vi "EF_GetFeaturesVectorPowerSpectrum.vi"(8 "error in (no error)":errorcluster, 11 "Array Of Waveforms in":waveform(dbl)[](array[waveform])) -> (0 "error out":errorcluster, 3 "Features Array out":dbl[][](array[numeric]))   [LabVIEW 2016, in "Feature Extraction.lvlib"]
uses:
  <vilib>/Analysis/2dsp.llb/Power Spectrum (DBL).vi
  Feature Extraction.lvlib
  <vilib>/Analysis/NI_AALPro.lvlib
panel:
  # "This VI is a part of BCI Design library, http://www.ru-bci.org \nCopyright © 2020, Sotnikov Peter, All rights reserved. License: GNU GPLv3"
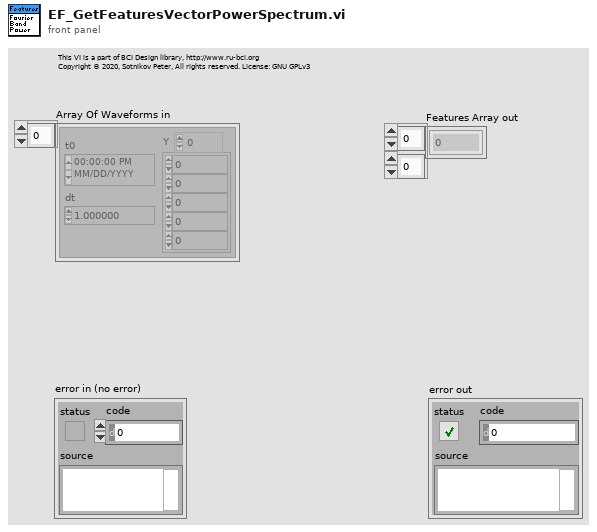
[diagram p1: front panel]
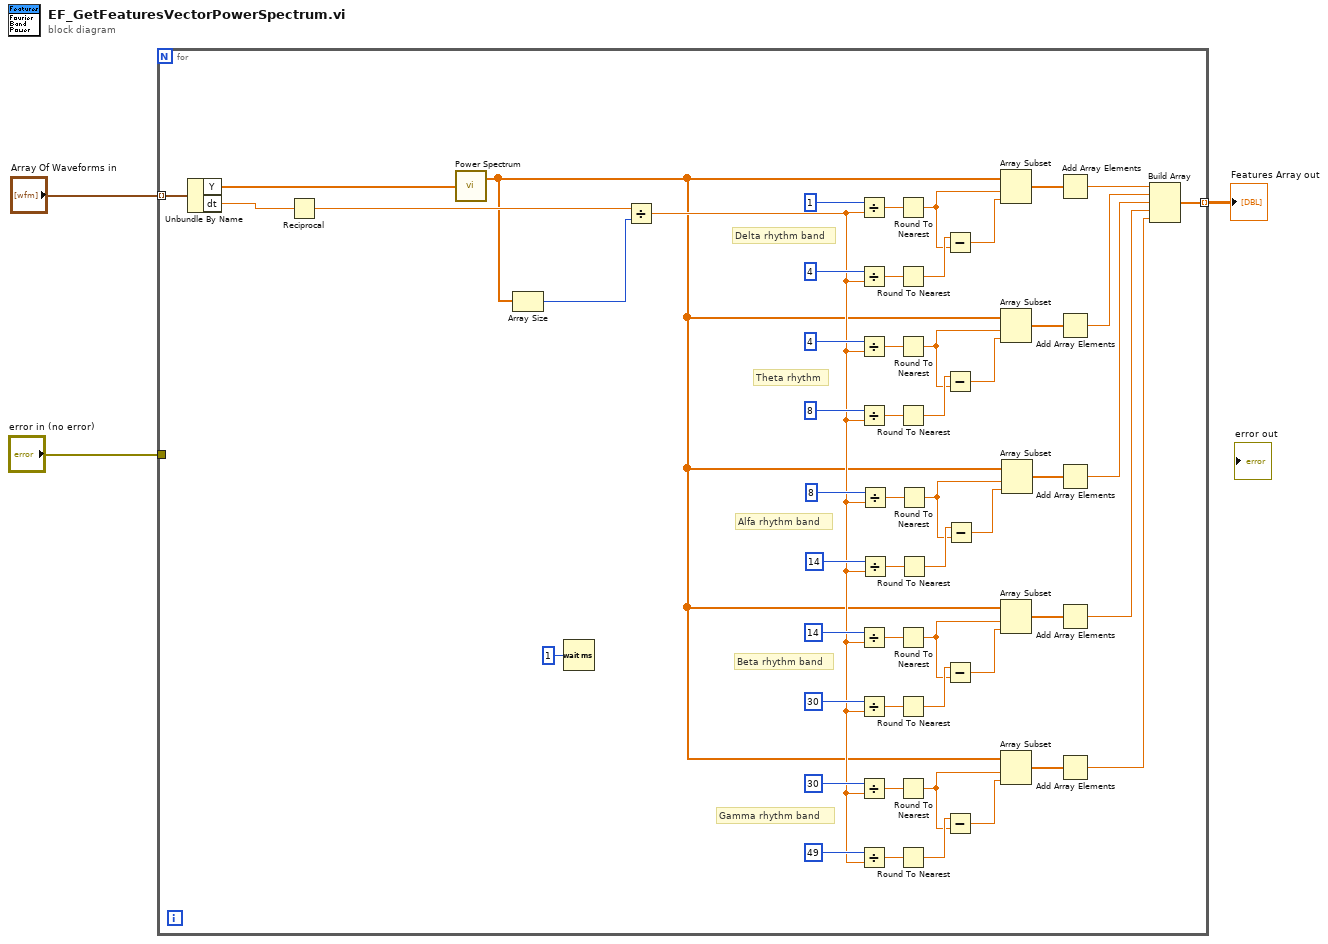
[diagram p0: block diagram]
diagram:
  n1 = for {
    tunnel: "Array Of Waveforms in" -> [w32] mode=indexing
    tunnel: "error in (no error)" -> [_]
    tunnel: [w5] -> w1 mode=indexing
    # "Gamma rhythm band"
    # "Beta rhythm band"
    # "Theta rhythm"
    # "Delta rhythm band"
    # "Alfa rhythm band"
    n2 = Unbundle By Name(w32) -> ("Y"=w4:dbl[], "dt"=w16:dbl)
    n3 = Reciprocal(x=w16) -> (1/x=w7:dbl)
    n4 = call-poly <vilib>:"Power Spectrum.vi"("X"=w4) -> ("Power Spectrum"=w6:dbl[])  [unwired: 1 out]
    n5 = Array Size(array=w6) -> (size(s)=w13:i32)
    n6 = Wait (ms)(milliseconds to wait=u32 1) -> ()  [unwired: 1 out]
    n7 = Divide(x=w7, y=w13) -> (x/y=w15:dbl)
    n8 = Divide(x=1, y=w15) -> (x/y=w57:dbl)
    n9 = Divide(x=4, y=w15) -> (x/y=w55:dbl)
    n10 = Divide(x=4, y=w15) -> (x/y=w52:dbl)
    n11 = Divide(x=8, y=w15) -> (x/y=w50:dbl)
    n12 = Divide(x=14, y=w15) -> (x/y=w42:dbl)
    n13 = Divide(x=30, y=w15) -> (x/y=w40:dbl)
    n14 = Divide(x=30, y=w15) -> (x/y=w37:dbl)
    n15 = Divide(x=49, y=w15) -> (x/y=w35:dbl)
    n16 = Divide(x=8, y=w15) -> (x/y=w47:dbl)
    n17 = Divide(x=14, y=w15) -> (x/y=w45:dbl)
    n18 = Round To Nearest(number=w57) -> (nearest integer value=w31:dbl)
    n19 = Round To Nearest(number=w55) -> (nearest integer value=w53:dbl)
    n20 = Round To Nearest(number=w52) -> (nearest integer value=w29:dbl)
    n21 = Round To Nearest(number=w50) -> (nearest integer value=w48:dbl)
    n22 = Round To Nearest(number=w42) -> (nearest integer value=w25:dbl)
    n23 = Round To Nearest(number=w40) -> (nearest integer value=w38:dbl)
    n24 = Round To Nearest(number=w37) -> (nearest integer value=w27:dbl)
    n25 = Round To Nearest(number=w35) -> (nearest integer value=w33:dbl)
    n26 = Round To Nearest(number=w47) -> (nearest integer value=w23:dbl)
    n27 = Round To Nearest(number=w45) -> (nearest integer value=w43:dbl)
    n28 = Subtract(x=w53, y=w31) -> (x-y=w30:dbl)
    n29 = Subtract(x=w48, y=w29) -> (x-y=w28:dbl)
    n30 = Subtract(x=w38, y=w25) -> (x-y=w24:dbl)
    n31 = Subtract(x=w33, y=w27) -> (x-y=w26:dbl)
    n32 = Subtract(x=w43, y=w23) -> (x-y=w17:dbl)
    n33 = Array Subset(array=w6, index=w31, length=w30) -> (w22:dbl[])
    n34 = Array Subset(array=w6, index=w29, length=w28) -> (w21:dbl[])
    n35 = Array Subset(array=w6, index=w25, length=w24) -> (w19:dbl[])
    n36 = Array Subset(array=w6, index=w27, length=w26) -> (w18:dbl[])
    n37 = Array Subset(array=w6, index=w23, length=w17) -> (w20:dbl[])
    n38 = Add Array Elements(numeric array=w22) -> (sum=w12:dbl)
    n39 = Add Array Elements(numeric array=w21) -> (sum=w11:dbl)
    n40 = Add Array Elements(numeric array=w20) -> (sum=w10:dbl)
    n41 = Add Array Elements(numeric array=w19) -> (sum=w9:dbl)
    n42 = Add Array Elements(numeric array=w18) -> (sum=w8:dbl)
    n43 = Build Array(w12, w11, w10, w9, w8) -> (w5:dbl[])
  }
  "Features Array out" <- w1
